vi "与主屏通信master.vi"() -> ()   [LabVIEW 2016, in "斯坦道多参数.lvlib"]
uses:
  <vilib>/NI/Modbus Library/API/Wrapper/Create TCP Master.vi
  <vilib>/NI/Modbus Library/API/master/Modbus Master.lvclass
  <vilib>/NI/Modbus Library/API/Wrapper/API Main.lvlib
  <vilib>/ptbypt/NI_PtbyPt.lvlib
panel:
  out "主屏启动命令":u16
  in  "registers to write":u16[](array[numeric])
  out "error out":errorcluster
  in  "停止":bool
  out "read values":u16[](array[numeric])
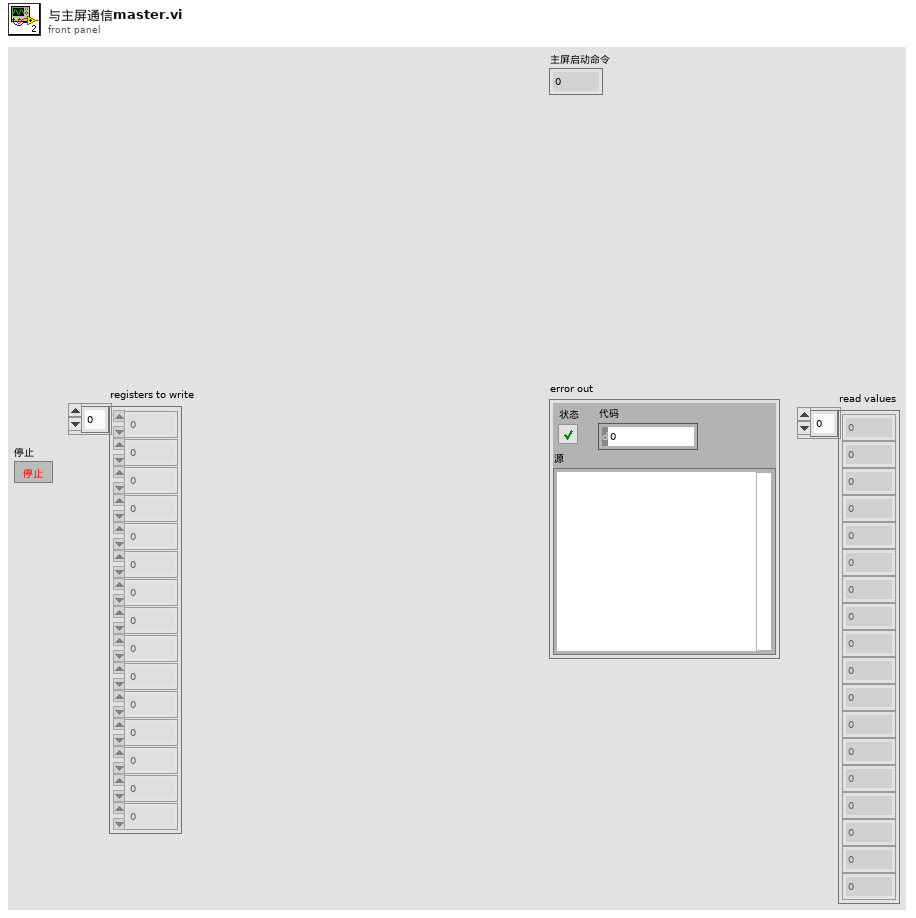
[diagram p1: front panel]
types:
  T1 = cluster{"数据保存间隔":dbl, "水温标样值":dbl, "pH标样值":dbl, "溶解氧标样值":dbl, "电导率标样值":dbl, "浊度标样值":dbl}
  T2 = enum32{"Bad", "Idle", "Run top level", "Running"}
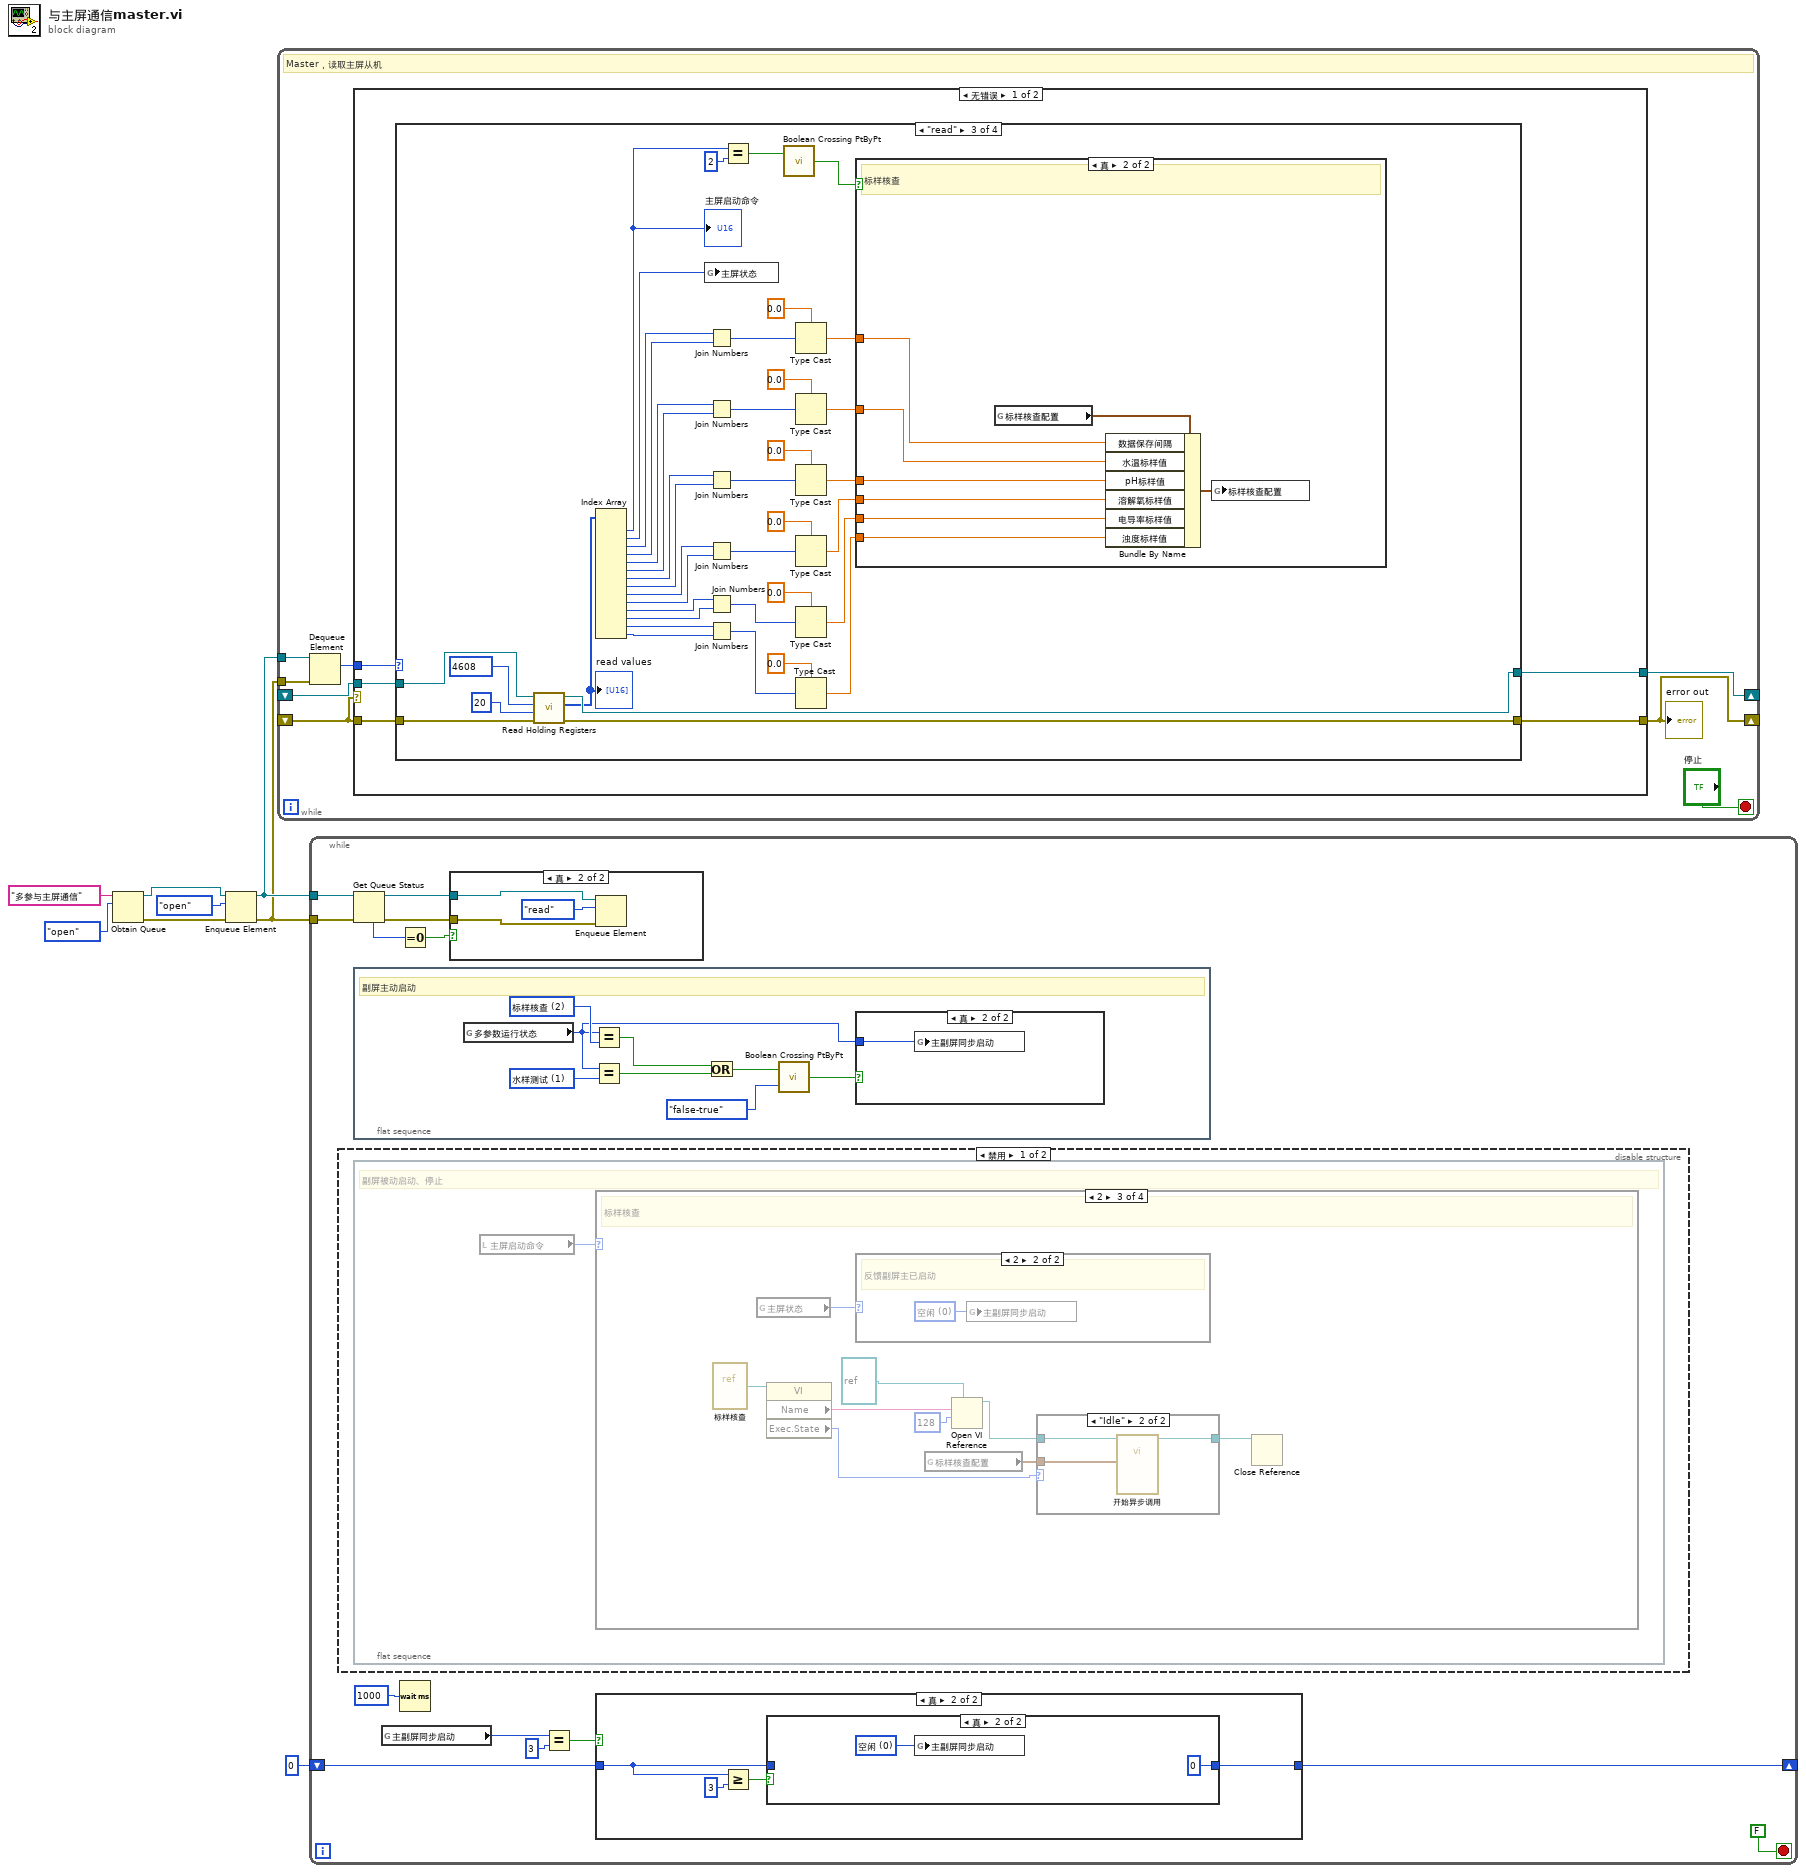
[diagram p0: block diagram]
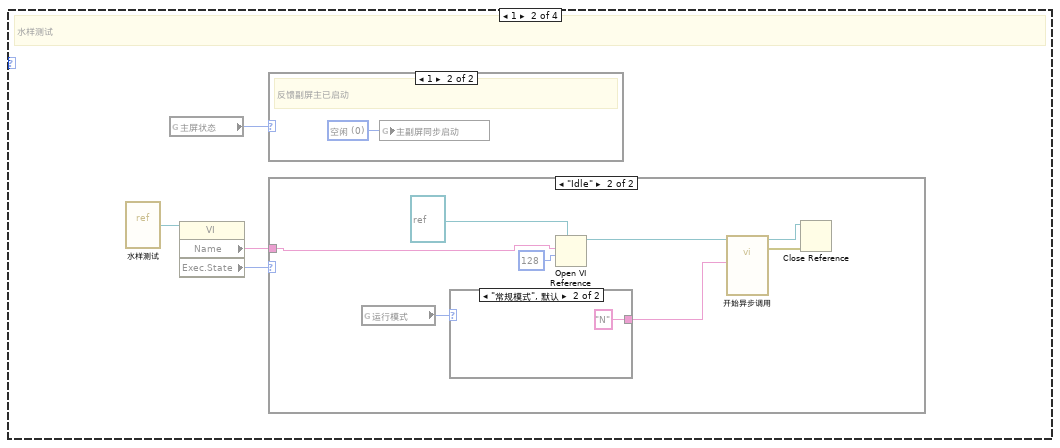
[diagram p3: hidden frame]
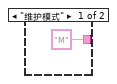
[diagram p6: hidden frame]
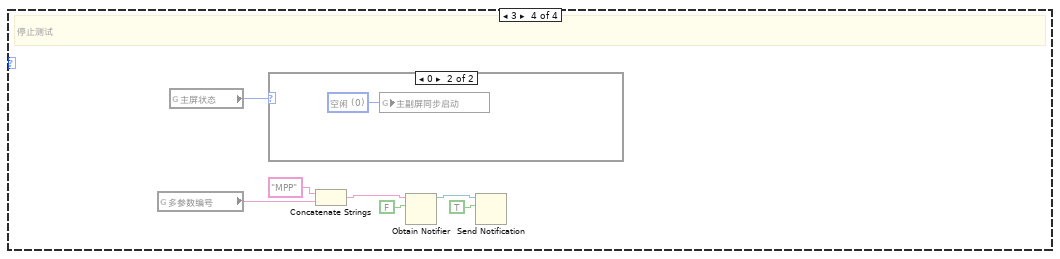
[diagram p9: hidden frame]
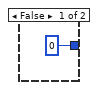
[diagram p12: hidden frame]
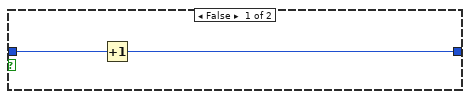
[diagram p13: hidden frame]
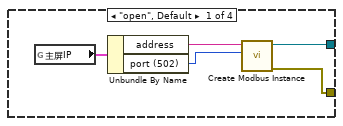
[diagram p16: hidden frame]
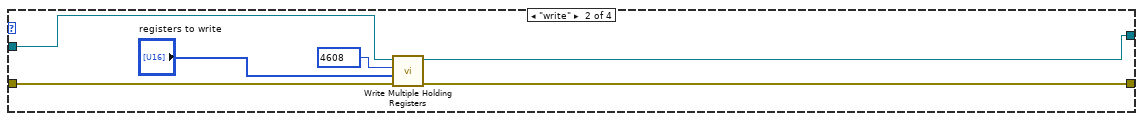
[diagram p17: hidden frame]
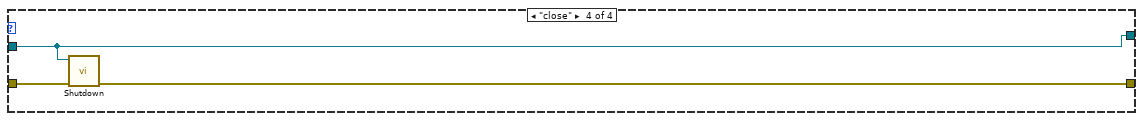
[diagram p19: hidden frame]
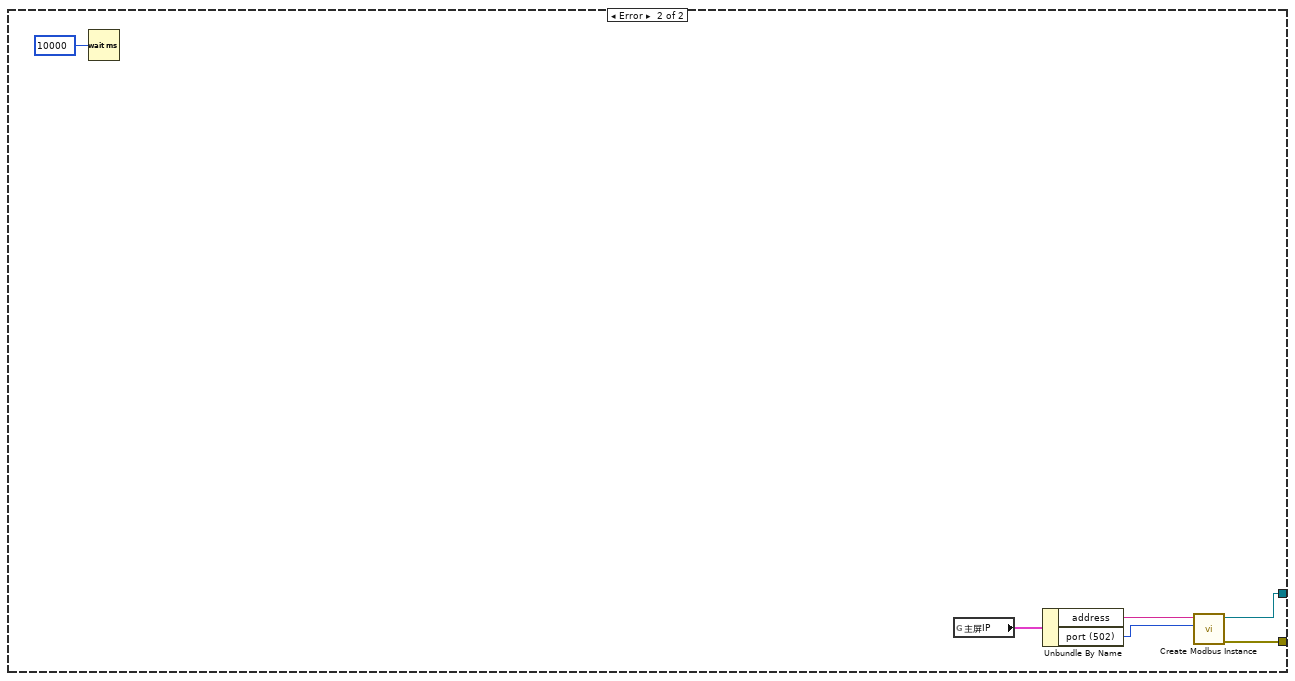
[diagram p20: hidden frame]
diagram:
  n1 = Obtain Queue(name (unnamed)="多参与主屏通信" ("名称（未命名）"), element data type=enum16{"open", "write", "read", "close"}."open") -> (queue out=w7:refnum<queue>, error out=w6:errorcluster)  [unwired: 3 in, 1 out]
  n2 = Enqueue Element(queue=w7, element=enum16{"open", "write", "read", "close"}."open", error in (no error)=w6) -> (queue out=w3:refnum<queue>, error out=w2:errorcluster)  [unwired: 1 in, 1 out]
  n3 = while {
    shift-right: [w13] -> _
    shift-left: _ -> [w15]
    shift-right: [w14] -> _
    shift-left: _ -> [w12]
    tunnel: w3 -> [w11]
    tunnel: w2 -> [w10]
    stop <- "停止" stop-if-true
    # "Master，读取主屏从机"
    n4 = Dequeue Element(queue=w11, error in (no error)=w10) -> (element=w9:enum16{"open", "write", "read", "close"})  [unwired: 1 in, 3 out]
    n5 = case shown="无错误" w12 {
      tunnel: w15 -> [w21 _]
      tunnel: w12 -> [w20 _]
      tunnel: [w19 w90] -> w14
      tunnel: [w18 w91] -> w13
      tunnel: w9 -> [w17 _]
      frame No Error {
        n6 = case shown="\"read\"" w17 {
          tunnel: w21 -> [_ w32 w74 w85]
          tunnel: w20 -> [_ w30 w71 w84]
          tunnel: [w25 w27 w70 w83] -> w19
          tunnel: [w26 w28 w69 w85] -> w18
          frame "open", Default {
            n7 = global read "多参数全局变量.vi" "主屏IP"() -> (w24:cluster{"address":string, "port (502)":u16})
            n8 = Unbundle By Name(w24) -> ("address"=w23:string, "port (502)"=w22:u16)
            n9 = call-poly <vilib>:"Create Modbus Instance.vi"("port (502)"=w22, "address"=w23) -> ("error out"=w25:errorcluster, "TCP master instance"=w26:refnum<class "Modbus Master.lvclass">)  [unwired: 8 in]
          }
          frame "write" {
            n10 = call-dynamic "Write Multiple Holding Registers.vi"("error in"=w30, "registers to write"="registers to write", "starting address"=u16 4608 ("write starting address"), "Modbus master in"=w32) -> ("error out"=w27:errorcluster, "Modbus master out"=w28:refnum<class "Modbus Master.lvclass">)  [unwired: 6 in]
          }
          frame "read" {
            n11 = call-dynamic "Read Holding Registers.vi"("error in"=w71, "number of inputs"=u16 20 ("read count"), "starting address"=u16 4608 ("write starting address"), "Modbus master in"=w74) -> ("error out"=w70:errorcluster, "register values"=w68:u16[], "Modbus master out"=w69:refnum<class "Modbus Master.lvclass">)  [unwired: 5 in]
            "read values" <- w68
            n12 = Index Array(array=w68) -> (element #1=w36:u16, element #2=w67:u16, element #3=w64:u16, element #4=w63:u16, element #5=w57:u16, element #6=w58:u16, element #7=w53:u16, element #8=w54:u16, element #9=w48:u16, element #10=w47:u16, element #11=w40:u16, element #12=w39:u16, element #13=w38:u16, element #14=w37:u16)  [unwired: 14 in]
            "主屏启动命令" <- w36
            n13 = global write "多参数全局变量.vi" "主屏状态"(w67) -> ()
            n14 = Join Numbers(hi=w64, lo=w63) -> ((hi.lo)=w65:u32)
            n15 = Join Numbers(hi=w57, lo=w58) -> ((hi.lo)=w60:u32)
            n16 = Join Numbers(hi=w53, lo=w54) -> ((hi.lo)=w55:u32)
            n17 = Join Numbers(hi=w48, lo=w47) -> ((hi.lo)=w50:u32)
            n18 = Join Numbers(hi=w40, lo=w39) -> ((hi.lo)=w45:u32)
            n19 = Join Numbers(hi=w38, lo=w37) -> ((hi.lo)=w43:u32)
            n20 = Equal?(x=w36, y=u16 2) -> (x = y?=w34:bool)
            n21 = call <vilib>:"Boolean Crossing PtByPt.vi"("input"=w34) -> ("crossing"=w33:bool)  [unwired: 2 in]
            n22 = Type Cast(type=sgl 0.0, x=w65) -> (*(type *) &x=w62:sgl)
            n23 = Type Cast(type=sgl 0.0, x=w60) -> (*(type *) &x=w59:sgl)
            n24 = Type Cast(type=sgl 0.0, x=w55) -> (*(type *) &x=w52:sgl)
            n25 = Type Cast(type=sgl 0.0, x=w50) -> (*(type *) &x=w49:sgl)
            n26 = Type Cast(type=sgl 0.0, x=w45) -> (*(type *) &x=w42:sgl)
            n27 = Type Cast(type=sgl 0.0, x=w43) -> (*(type *) &x=w41:sgl)
            n28 = case shown="真" w33 {
              tunnel: w62 -> [_ w80]
              tunnel: w59 -> [_ w79]
              tunnel: w52 -> [_ w78]
              tunnel: w49 -> [_ w77]
              tunnel: w42 -> [_ w76]
              tunnel: w41 -> [_ w75]
              frame False {
              }
              frame True {
                # "标样核查"
                n29 = global read "断电保存变量.vi" "标样核查配置"() -> (w82:T1)
                n30 = Bundle By Name(cluster=w82, "数据保存间隔"=w80, "水温标样值"=w79, "pH标样值"=w78, "溶解氧标样值"=w77, "电导率标样值"=w76, "浊度标样值"=w75) -> (w81:T1)
                n31 = global write "断电保存变量.vi" "标样核查配置"(w81) -> ()
              }
            }
          }
          frame "close" {
            n32 = call-dynamic "Shutdown.vi"("error in"=w84, "Modbus master in"=w85) -> ("error out"=w83:errorcluster)  [unwired: 9 in]
          }
        }
      }
      frame Error {
        n33 = Wait (ms)(milliseconds to wait=u32 10000 ("等待时间（毫秒）")) -> ()  [unwired: 1 out]
        n34 = global read "多参数全局变量.vi" "主屏IP"() -> (w88:cluster{"address":string, "port (502)":u16})
        n35 = Unbundle By Name(w88) -> ("address"=w87:string, "port (502)"=w86:u16)
        n36 = call-poly <vilib>:"Create Modbus Instance.vi"("port (502)"=w86, "address"=w87) -> ("error out"=w90:errorcluster, "TCP master instance"=w91:refnum<class "Modbus Master.lvclass">)  [unwired: 8 in]
      }
    }
    "error out" <- w14
  }
  n37 = while {
    tunnel: w3 -> [w104]
    tunnel: w2 -> [w103]
    shift-right: [w92] -> _
    shift-left: u32 0 ("等待时间（毫秒）") -> [w93]
    stop <- FALSE stop-if-true
    n38 = disable-structure shown="禁用" {
      frame Disabled {
        n39 = flat-sequence {
          frame #0 {
            # "副屏被动启动、停止"
            n40 = local read "主屏启动命令"() -> (w105:u16)
            n41 = case shown="2" w105 {
              frame 0, Default {
              }
              frame 1 {
                # "水样测试"
                n42 = vi-ref "水样测试.vi"() -> (w109:refnum<vi>)
                n43 = global read "多参数全局变量.vi" "主屏状态"() -> (w106:u16)
                n44 = property class="VI"(reference=w109) -> ("Name"=w107:string, "Exec.State"=w108:T2)  [unwired: 1 in, 2 out]
                n45 = case shown="1" w106 {
                  frame 0, Default {
                  }
                  frame 1 {
                    w110 = u16 0 items=["空闲", "水样测试", "标样核查", "停止"] ("主副屏同步启动")
                    # "反馈副屏主已启动"
                    n46 = global write "多参数全局变量.vi" "主副屏同步启动"(w110) -> ()
                  }
                }
                n47 = case shown="\"Idle\"" w108 {
                  tunnel: w107 -> [_ w115]
                  frame "Bad", Default {
                  }
                  frame "Idle" {
                    n48 = global read "多参数全局变量.vi" "运行模式"() -> (w113:enum16{"维护模式", "常规模式", "应急模式", "质控模式"})
                    n49 = case shown="\"常规模式\", 默认" w113 {
                      tunnel: ["M" ("数据标记表") "N" ("数据标记表")] -> w112
                      frame "维护模式" {
                      }
                      frame "常规模式", Default {
                      }
                    }
                    n50 = Open VI Reference(type specifier VI Refnum (for type only)=refnum<vi> refnum, vi path=w115, options=128 ("选项")) -> (vi reference=w116:refnum<vi>)  [unwired: 3 in, 1 out]
                    n51 = call-by-ref "开始异步调用"(reference=w116, "数据标记表"=w112) -> (reference out=w117:refnum<vi>, error out=w118:errorcluster)  [unwired: 12 in]
                    n52 = Close Reference(reference=w117, error in (no error)=w118) -> ()  [unwired: 1 out]
                  }
                }
              }
              frame 2 {
                # "标样核查"
                n53 = vi-ref "标样核查.vi"() -> (w128:refnum<vi>)
                n54 = global read "多参数全局变量.vi" "主屏状态"() -> (w129:u16)
                n55 = property class="VI"(reference=w128) -> ("Name"=w124:string, "Exec.State"=w126:T2)  [unwired: 1 in, 2 out]
                n56 = case shown="2" w129 {
                  frame 0, Default {
                  }
                  frame 2 {
                    w130 = u16 0 items=["空闲", "水样测试", "标样核查", "停止"] ("主副屏同步启动")
                    # "反馈副屏主已启动"
                    n57 = global write "多参数全局变量.vi" "主副屏同步启动"(w130) -> ()
                  }
                }
                n58 = global read "断电保存变量.vi" "标样核查配置"() -> (w122:T1)
                n59 = Open VI Reference(type specifier VI Refnum (for type only)=refnum<vi> refnum, vi path=w124, options=128 ("选项")) -> (vi reference=w123:refnum<vi>)  [unwired: 3 in, 1 out]
                n60 = case shown="\"Idle\"" w126 {
                  tunnel: [w131 w134] -> w127
                  tunnel: w123 -> [w131 w133]
                  tunnel: w122 -> [_ w132]
                  frame "Bad", Default {
                  }
                  frame "Idle" {
                    n61 = call-by-ref "开始异步调用"(reference=w133, "标样核查配置"=w132) -> (reference out=w134:refnum<vi>)  [unwired: 12 in, 1 out]
                  }
                }
                n62 = Close Reference(reference=w127) -> ()  [unwired: 1 in, 1 out]
              }
              frame 3 {
                # "停止测试"
                n63 = global read "多参数全局变量.vi" "多参数编号"() -> (w138:string)
                n64 = global read "多参数全局变量.vi" "主屏状态"() -> (w135:u16)
                n65 = case shown="0" w135 {
                  frame 1, Default {
                  }
                  frame 0 {
                    w142 = u16 0 items=["空闲", "水样测试", "标样核查", "停止"] ("主副屏同步启动")
                    n66 = global write "多参数全局变量.vi" "主副屏同步启动"(w142) -> ()
                  }
                }
                n67 = Concatenate Strings("MPP" ("名称（未命名）"), w138) -> (w139:string)
                n68 = Obtain Notifier(name (unnamed)=w139, notification data type=FALSE) -> (notifier out=w136:refnum<notifier>)  [unwired: 2 in, 2 out]
                n69 = Send Notification(notification=TRUE ("通知"), notifier=w136) -> ()  [unwired: 1 in, 2 out]
              }
            }
          }
        }
      }
      frame Enabled {
      }
    }
    n70 = Get Queue Status(queue=w104, error in (no error)=w103) -> (queue out=w100:refnum<queue>, error out=w99:errorcluster, # elements in queue=w102:i32)  [unwired: 1 in, 5 out]
    n71 = flat-sequence {
      frame #0 {
        w154 = u16 2 items=["空闲", "水样测试", "标样核查"] ("多参数运行状态")
        w157 = u16 1 items=["空闲", "水样测试", "标样核查"] ("多参数运行状态")
        # "副屏主动启动"
        n72 = global read "多参数全局变量.vi" "多参数运行状态"() -> (w153:u16)
        n73 = Equal?(x=w153, y=w154) -> (x = y?=w152:bool)
        n74 = Equal?(x=w153, y=w157) -> (x = y?=w158:bool)
        n75 = Or(x=w152, y=w158) -> (x .or. y?=w155:bool)
        n76 = call <vilib>:"Boolean Crossing PtByPt.vi"("direction"=enum16{"either", "false-true", "true-false"}."false-true", "input"=w155) -> ("crossing"=w156:bool)  [unwired: 1 in]
        n77 = case shown="真" w156 {
          tunnel: w153 -> [_ w160]
          frame False {
          }
          frame True {
            n78 = global write "多参数全局变量.vi" "主副屏同步启动"(w160) -> ()
          }
        }
      }
    }
    n79 = global read "多参数全局变量.vi" "主副屏同步启动"() -> (w96:u16)
    n80 = Equal To 0?(x=w102) -> (x = 0?=w98:bool)
    n81 = Wait (ms)(milliseconds to wait=u32 1000 ("等待时间（毫秒）")) -> ()  [unwired: 1 out]
    n82 = case shown="真" w98 {
      tunnel: w100 -> [_ w162]
      tunnel: w99 -> [_ w161]
      frame False {
      }
      frame True {
        n83 = Enqueue Element(queue=w162, element=enum16{"open", "write", "read", "close"}."read", error in (no error)=w161) -> ()  [unwired: 1 in, 3 out]
      }
    }
    n84 = Equal?(x=w96, y=u16 3) -> (x = y?=w94:bool)
    n85 = case shown="真" w94 {
      tunnel: w93 -> [_ w146]
      tunnel: [u32 0 w147] -> w92
      frame False {
      }
      frame True {
        n86 = Greater Or Equal?(x=w146, y=u32 3) -> (x >= y?=w144:bool)
        n87 = case shown="真" w144 {
          tunnel: [w149 u32 0] -> w147
          tunnel: w146 -> [w148 _]
          frame False {
            n88 = Increment(x=w148) -> (x+1=w149:u32)
          }
          frame True {
            w151 = u16 0 items=["空闲", "水样测试", "标样核查", "停止"] ("主副屏同步启动")
            n89 = global write "多参数全局变量.vi" "主副屏同步启动"(w151) -> ()
          }
        }
      }
    }
  }
